vi "Xml_Save_Timing_Table.vi"(8 "error in (no error)":errorcluster, 11 "Refnum Clust":refnum<vi>) -> (0 "error out":errorcluster, 3 "XML String Out":string)   [LabVIEW 2018]
doc: "This VI saves the TIMING Table parameters to XML format."
uses:
  controls/TIMING_Table.ctl
  controls/TIMING_Mandatory_Items.ctl
  controls/TIMING_Optional_Items.ctl
panel:
  in  "TIMING Table":T1={"Mandatory Items"={"Script Name"="", "GINI Time Period"=100.0, "HSDIO Delay"=60.0, "Shutter Duration before"=50000.0, "Shutter Duration after"=50000.0, "Filter Tau"=2.0, "Emtyping Duration"=1000.0}, "Optional Items"={"Eject"=0, "Acq"=0, "Excit"=0, "Gas"=0, "Laser"=0, "Lamp"=0}, "Times Table"=[["Excit1", "name", "Swift", "0.5", "1200", "70", "150", "550", "0", "0", "0"]]} {"Optional Items"."Laser" min=0 max=3; "Optional Items"."Gas" min=0 max=5; "Mandatory Items"."GINI Time Period" min=100000.0 max=1000000.0 format="%#_7g"; "Mandatory Items"."Shutter Duration after" min=2.0 max=100000.0; "Mandatory Items"."HSDIO Delay" min=0.0 max=100.0; "Mandatory Items"."Shutter Duration before" min=2.0 max=100000.0; "Mandatory Items"."Filter Tau" min=1000.0 max=2000.0; "Mandatory Items"."Emtyping Duration" min=2.0 format="%#_8g"}
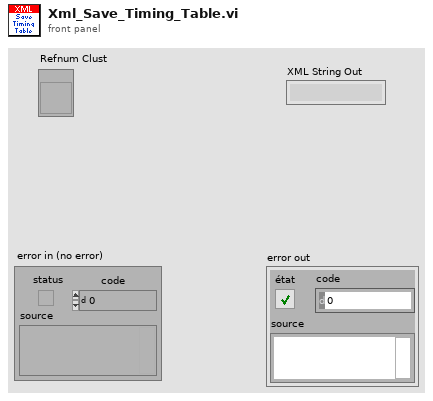
[diagram p1: front panel]
types:
  T1 = typedef "TIMING_Table.ctl" = cluster{"Mandatory Items":T2, "Optional Items":T3, "Times Table":string[][]}
  T2 = typedef "TIMING_Mandatory_Items.ctl" = cluster{"Script Name":string, "GINI Time Period":dbl, "HSDIO Delay":dbl, "Shutter Duration before":dbl, "Shutter Duration after":dbl, "Filter Tau":dbl, "Emtyping Duration":dbl}
  T3 = typedef "TIMING_Optional_Items.ctl" = cluster{"Eject":u32, "Acq":i32, "Excit":u32, "Gas":i32, "Laser":i32, "Lamp":i32}
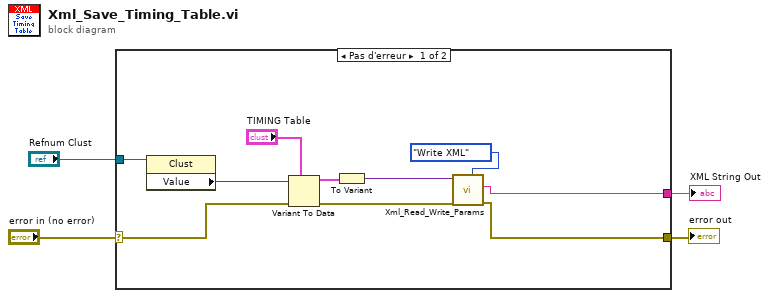
[diagram p0: block diagram]
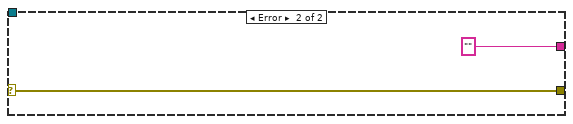
[diagram p2: hidden frame]
diagram:
  n1 = case shown="Pas d'erreur" "error in (no error)" {
    selector: "error in (no error)" -> [w14 w16]
    tunnel: [w13 w16] -> w3
    tunnel: [w12 "" ("XML String Out")] -> w2
    tunnel: "Refnum Clust" -> [w7 _]
    frame No Error {
      n2 = property class="Clust"(reference=w7) -> ("Value"=w8:variant)  [unwired: 1 in, 2 out]
      n3 = Variant To Data(error in=w14, type="TIMING Table", Variant=w8) -> (data=w6:T1, error out=w9:errorcluster)
      n4 = To Variant(anything=w6) -> (Variant=w11:variant)
      n5 = call "Xml_Read_Write_Params.vi"("Variant"=w11, "error in (no error)"=w9, "Command"=enum16{"Read XML", "Set", "Get", "Write XML"}."Write XML") -> ("XML String Out"=w12:string, "error out"=w13:errorcluster)  [unwired: 4 in, 1 out]
    }
    frame Error {
    }
  }
  "error out" <- w3
  "XML String Out" <- w2
